vi "getLoggerRef.vi"(9 "error in (no error)":errorcluster) -> (1 "error out":errorcluster, 3 "Logger Ref":refnum<data-value>)   [LabVIEW 2017, in "Error Log.lvlib" / "Logger.lvclass"]
uses:
  Logger.lvclass
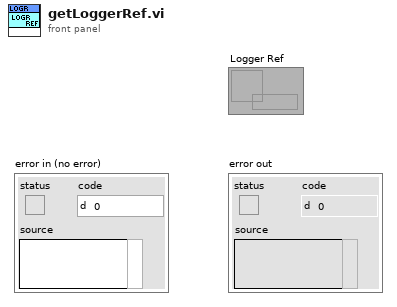
[diagram p1: front panel]
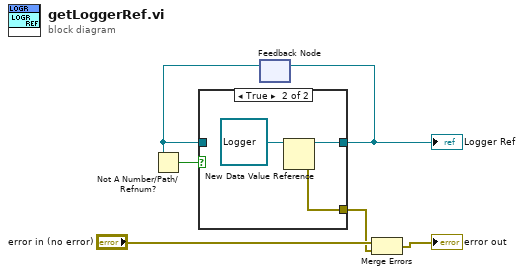
[diagram p0: block diagram]
diagram:
  n1 = feedback #1() -> (w4:refnum<data-value>)  [unwired: 1 in]
  n2 = Not A Number/Path/Refnum?(number/path/refnum=w4) -> (NaN/Path/Refnum?=w5:bool)
  n3 = case shown="True" w5 {
    tunnel: [w7 w10] -> w6
    tunnel: [_ w9] -> w1
    tunnel: w4 -> [w7 _]
    frame False {
    }
    frame True {
      n4 = New Data Value Reference(data value=refnum<class "Logger.lvclass"> refnum ("Logger in")) -> (data value reference=w10:refnum<data-value>, error out=w9:errorcluster)  [unwired: 1 in]
    }
  }
  "Logger Ref" <- w6
  n5 = feedback-in #1(w6) -> ()
  n6 = Merge Errors("error in (no error)", w1) -> (→"error out":errorcluster)
